vi "EEI EXP10.vi"() -> ()   [LabVIEW 2020]
panel:
  out "mp":dbl
  in  "l":dbl
  in  "m":dbl
  in  "ir":dbl
  out "output variable":dbl
  in  "input variable 3":dbl
  in  "input variable 2":dbl
  in  "input variable":dbl
  out "current time":timestamp
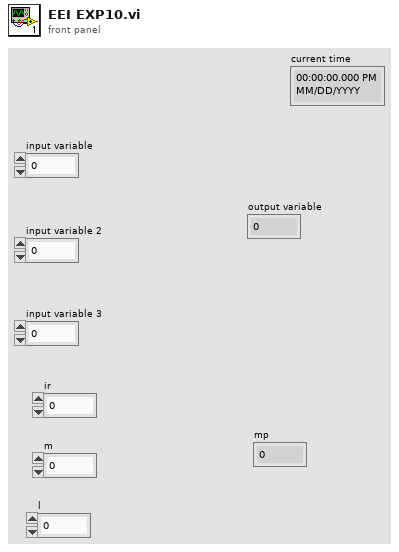
[diagram p1: front panel]
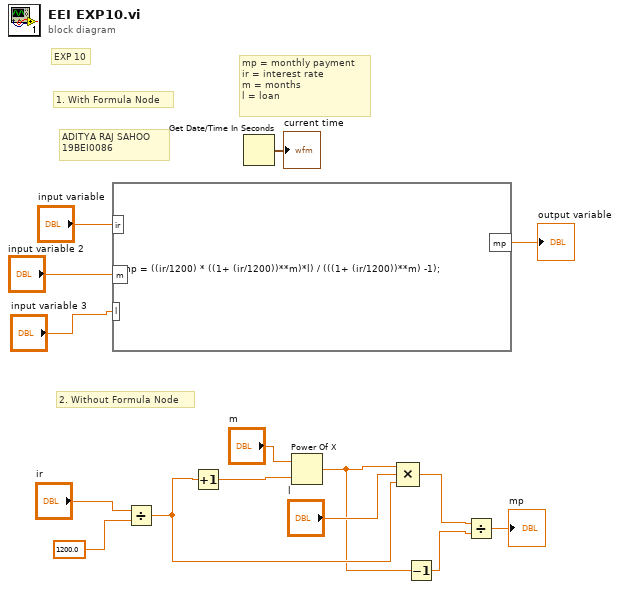
[diagram p0: block diagram]
diagram:
  # "2. Without Formula Node"
  # "mp = monthly payment\nir = interest rate\nm = months\nl = loan"
  # "1. With Formula Node"
  # "EXP 10"
  # "ADITYA RAJ SAHOO\n19BEI0086"
  n1 = formula code="mp = ((ir/1200) * ((1+ (ir/1200))**m)*l) / (((1+ (ir/1200))**m) -1);"("ir"="input variable", "m"="input variable 2", "l"="input variable 3") -> ("mp"=→"output variable":dbl)
  n2 = Divide(x="ir", y=1200.0) -> (x/y=w5:dbl)
  n3 = Increment(x=w5) -> (x+1=w8:dbl)
  n4 = Get Date/Time In Seconds() -> (seconds since 1Jan1904=→"current time":timestamp)
  n5 = Power Of X(1:w8, 2:"m") -> (0:w4:dbl)
  n6 = Compound Arithmetic op=MULTIPLY(w4, "l", w5) -> (w3:dbl)
  n7 = Decrement(x=w4) -> (x-1=w2:dbl)
  n8 = Divide(x=w3, y=w2) -> (x/y=→"mp":dbl)
